vi "RT_Create_RT_FIFOs.vi"(8 "error in (no error)":errorcluster) -> (0 "error out":errorcluster, 2 "Analog RT FIFO":refnum<k33>, 3 "Count RT FIFO":refnum<k33>)   [LabVIEW 2020]
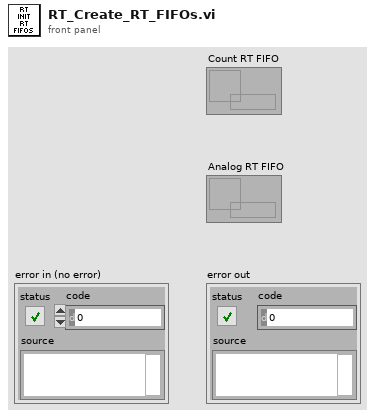
[diagram p1: front panel]
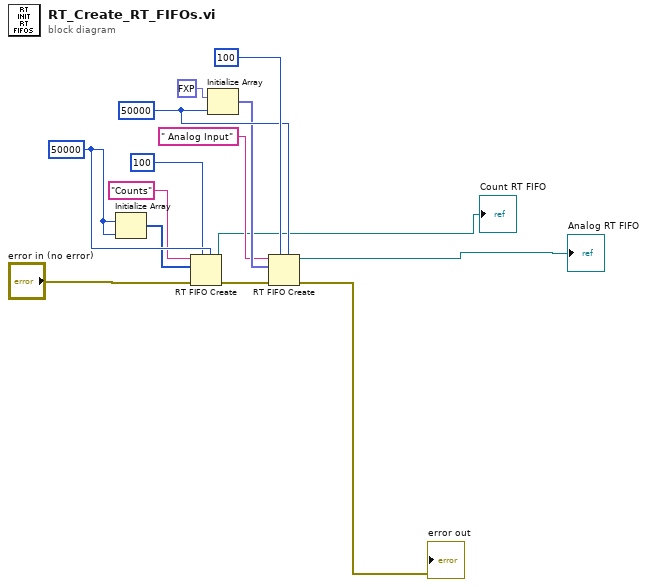
[diagram p0: block diagram]
diagram:
  w10 = 50000
  w11 = 50000 ("dimension size")
  n1 = Initialize Array(w10, w10) -> (w9:i32[])
  n2 = RT FIFO Create(0:"Counts" ("name (unnamed)"), 1:w9, 3:"error in (no error)", 4:u32 100 ("size (10)"), 6:w10) -> (8:→"Count RT FIFO":refnum<k33>, 11:w7:errorcluster)  [unwired: 3 in, 1 out]
  n3 = Initialize Array(fxp<+/-,17,5> 0.0, w11) -> (w6:fxp<+/-,17,5>[])
  n4 = RT FIFO Create(0:" Analog Input" ("name (unnamed)"), 1:w6, 3:w7, 4:u32 100 ("size (10)"), 6:w11) -> (8:→"Analog RT FIFO":refnum<k33>, 11:→"error out":errorcluster)  [unwired: 3 in, 1 out]
